vi "Main Panel.vi"() -> ()   [LabVIEW 2011]
uses:
  <vilib>/userdefined/High Color/IMAQdx.ctl
  <vilib>/vision/driver/NI_Vision_Acquisition_Software.lvlib
panel:
  out "Key Switch":bool
  out "Door Open":bool
  out "Flow Tank":dbl(slide) scale=0.0..100.0
  out "LCD Display":string
  out "Pump Irrigiation":bool
  out "Irrigation Empty Water":bool
  out "Hot Water On/Off?":bool
  out "AC/Heater On/Off?":bool
  out "What time you will be back?":dbl format="%#g"
  in  "STORE INFORMATIOn":bool
  out "Room2 Voice Recog":bool
  out "Room1 Voice Recog":bool
  out "Hot Water":bool
  out "Light Room2":bool
  out "Light Room1":bool
  in  "Hot Water":bool
  in  "Light Room2":bool
  in  "Light Room1":bool
  out "Manual AC Heater":bool
  in  "Manual Ac Heater":bool
  out "Fire Alarm":bool
  out "Manual Curtain":bool
  out "Curtain Open":bool
  out "Curtain close":bool
  in  "Close Curtain":bool
  in  "Open Curtain":bool
  in  "Manual Curtain":bool
  out "date":string
  out "time":string
  out "Solar Pos2":bool
  out "Solar Pos1":bool
  out "Light Intensity Pos2":dbl(knob) scale=0.0..100.0
  out "Light Intensity Pos1":dbl(knob) scale=0.0..100.0
  out "Water Temperature":dbl(slide) scale=0.0..100.0
  out "Temperature Inside":dbl(slide) scale=0.0..100.0
  out "Entree Light":bool
  out "RGB Door Led":bool
  out "Alarm Led":bool
  out "Low Level Water":bool
  out "Thief Alarm":bool
  out "Motion Detected":bool
  out "Dryer":bool
  out "Washing Machine":bool
  out "Heater":bool
  out "AC":bool
  in  "Restart Alarm":bool
  in  "Dryer":bool
  in  "AC":bool
  in  "Heater":bool
  in  "Washing Machine":bool
  out "WebCam":T1(plugin-control)
  in  "Exit":bool
  in  "Acess":bool
  out "Dor Lock/Unlock":bool
  in  "1":bool
  in  "2":bool
  in  "3":bool
  in  "4":bool
  in  "5":bool
  in  "6":bool
  in  "7":bool
  in  "8":bool
  in  "9":bool
  in  "0":bool
  out "Current":i32
  in  "0 2":bool
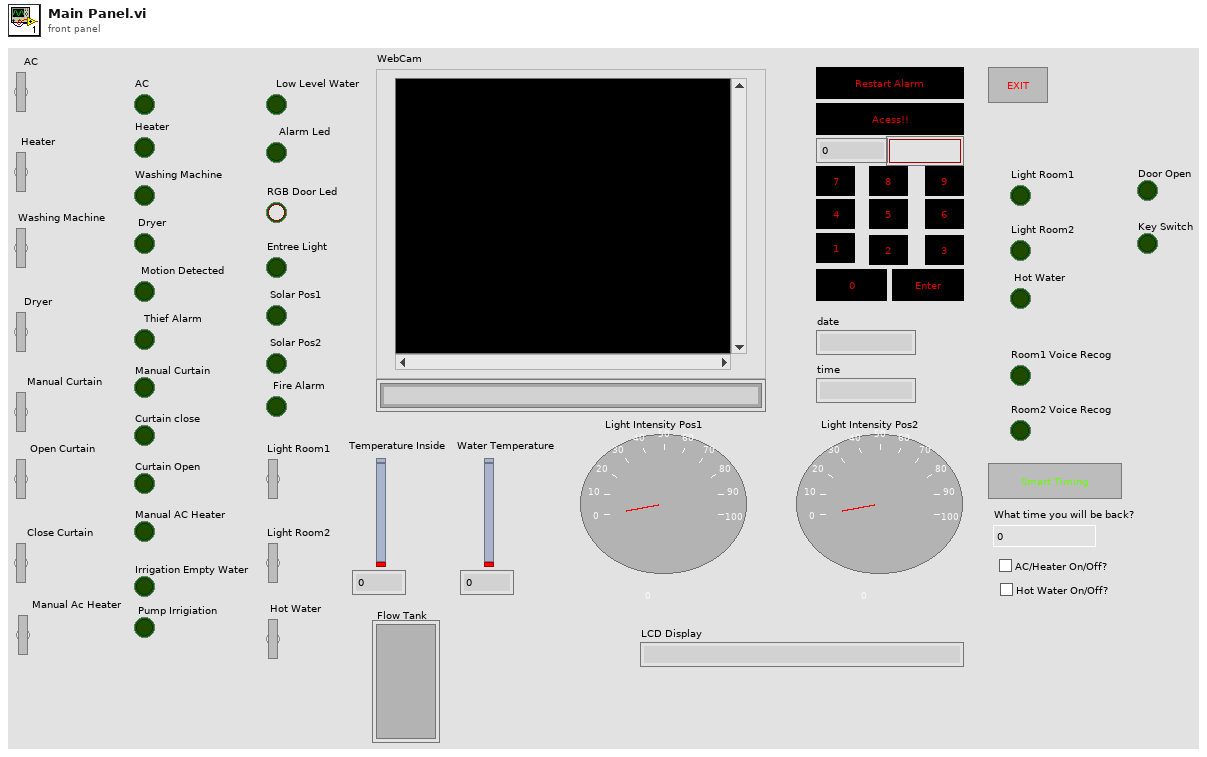
[diagram p1: front panel]
types:
  T1 = typedef "IMAQ Image.ctl" = refnum<image>
  T2 = typedef "IMAQdx.ctl" = refnum<k21>
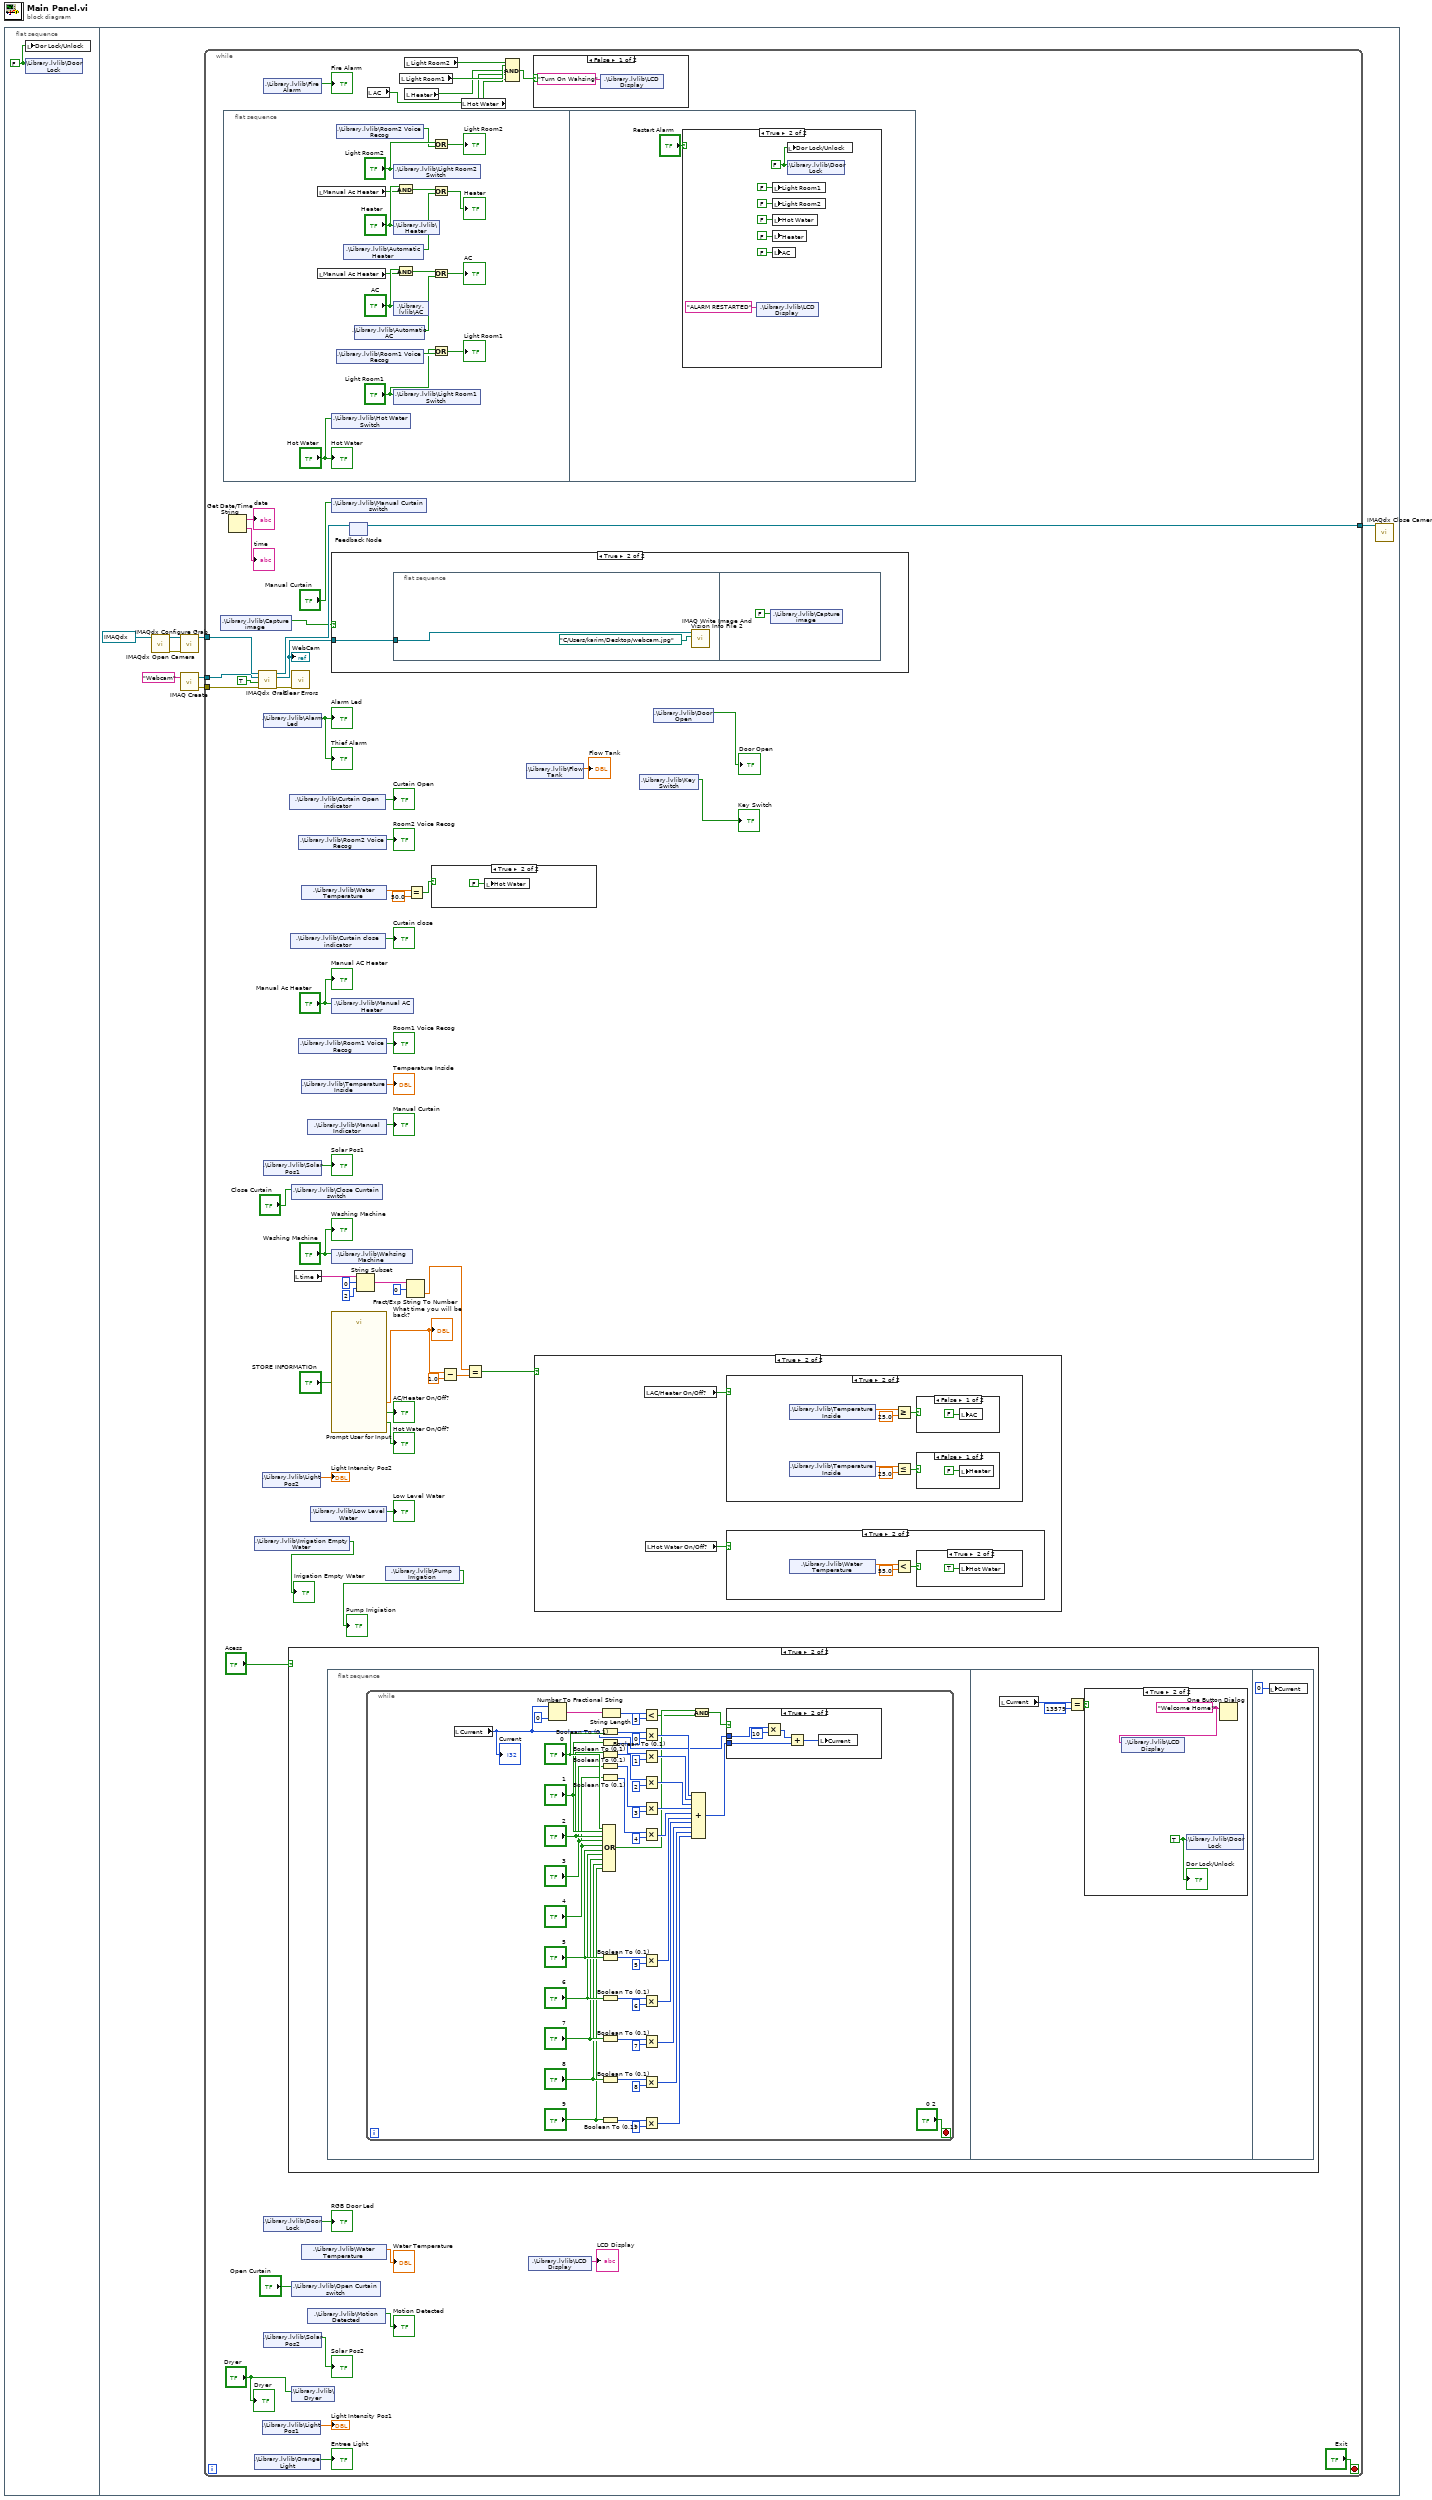
[diagram p0: block diagram]
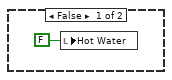
[diagram p5: hidden frame]
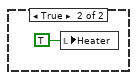
[diagram p7: hidden frame]
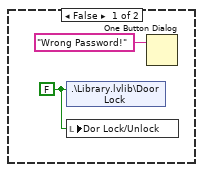
[diagram p13: hidden frame]
diagram:
  n1 = flat-sequence {
    frame #0 {
      w1 = FALSE ("Boolean")
      n2 = local write "Dor Lock/Unlock"(w1) -> ()
      n3 = shared-variable ".\\Library.lvlib\\Door Lock"(w1) -> ()  [unwired: 1 in, 1 out]
    }
    frame #1 {
      n4 = call <vilib>:"IMAQdx Open Camera.vi"("Session In"=T2 "cam0") -> ("error out"=w3:errorcluster, "Session Out"=w4:T2)  [unwired: 9 in]
      n5 = call <vilib>:"IMAQdx Configure Grab.vi"("error in"=w3, "Session In"=w4) -> ("Session Out"=w6:T2)  [unwired: 8 in, 1 out]
      n6 = call "IMAQ Create"("Image Name"="Webcam") -> ("New Image"=w5:T1, "error out"=w9:errorcluster)  [unwired: 4 in]
      n7 = while {
        tunnel: w5 -> [w69]
        tunnel: w6 -> [w72]
        tunnel: [w70] -> w7
        tunnel: w9 -> [w73]
        stop <- "Exit" stop-if-true
        n8 = shared-variable ".\\Library.lvlib\\Capture image"() -> (w63:bool)  [unwired: 1 in, 1 out]
        n9 = flat-sequence {
          frame #0 {
            n10 = local read "Manual Ac Heater"() -> (w93:bool)
            n11 = local read "Manual Ac Heater"() -> (w96:bool)
            n12 = shared-variable ".\\Library.lvlib\\Hot Water Switch"("Hot Water") -> ()  [unwired: 1 in, 1 out]
            n13 = shared-variable ".\\Library.lvlib\\Room2 Voice Recog"() -> (w104:bool)  [unwired: 1 in, 1 out]
            n14 = shared-variable ".\\Library.lvlib\\Room1 Voice Recog"() -> (w108:bool)  [unwired: 1 in, 1 out]
            n15 = shared-variable ".\\Library.lvlib\\Automatic Heater"() -> (w98:bool)  [unwired: 1 in, 1 out]
            n16 = shared-variable ".\\Library.lvlib\\Automatic AC"() -> (w101:bool)  [unwired: 1 in, 1 out]
            n17 = shared-variable ".\\Library.lvlib\\Light Room2 Switch"("Light Room2") -> ()  [unwired: 1 in, 1 out]
            n18 = shared-variable ".\\Library.lvlib\\Heater"("Heater") -> ()  [unwired: 1 in, 1 out]
            n19 = shared-variable ".\\Library.lvlib\\AC"("AC") -> ()  [unwired: 1 in, 1 out]
            n20 = shared-variable ".\\Library.lvlib\\Light Room1 Switch"("Light Room1") -> ()  [unwired: 1 in, 1 out]
            n21 = And(x="Heater", y=w93) -> (x .and. y?=w92:bool)
            n22 = And(x="AC", y=w96) -> (x .and. y?=w95:bool)
            n23 = Or(x="Light Room2", y=w104) -> (x .or. y?=→"Light Room2":bool)
            n24 = Or(x=w92, y=w98) -> (x .or. y?=→"Heater":bool)
            n25 = Or(x=w95, y=w101) -> (x .or. y?=→"AC":bool)
            n26 = Or(x="Light Room1", y=w108) -> (x .or. y?=→"Light Room1":bool)
            "Hot Water" <- "Hot Water"
          }
          frame #1 {
            n27 = case shown="True" "Restart Alarm" {
              frame False {
              }
              frame True {
                w116 = FALSE ("Boolean")
                n28 = shared-variable ".\\Library.lvlib\\LCD Display"("ALARM RESTARTED" ("LCD Display")) -> ()  [unwired: 1 in, 1 out]
                n29 = local write "Light Room1"(FALSE ("Light Room1")) -> ()
                n30 = local write "Light Room2"(FALSE ("Light Room2")) -> ()
                n31 = local write "Hot Water"(FALSE ("Hot Water")) -> ()
                n32 = local write "Heater"(FALSE ("Heater")) -> ()
                n33 = local write "AC"(FALSE ("AC")) -> ()
                n34 = local write "Dor Lock/Unlock"(w116) -> ()
                n35 = shared-variable ".\\Library.lvlib\\Door Lock"(w116) -> ()  [unwired: 1 in, 1 out]
              }
            }
          }
        }
        n36 = Get Date/Time String() -> (date string=→"date":string, time string=→"time":string)  [unwired: 3 in]
        n37 = shared-variable ".\\Library.lvlib\\Irrigation Empty Water"() -> (→"Irrigation Empty Water":bool)  [unwired: 1 in, 1 out]
        n38 = shared-variable ".\\Library.lvlib\\Orange Light"() -> (→"Entree Light":bool)  [unwired: 1 in, 1 out]
        n39 = call <vilib>:"IMAQdx Grab.vi"("error in"=w73, "Wait for Next Buffer? (Yes)"=TRUE, "Image In"=w69, "Session In"=w72) -> ("error out"=w64:errorcluster, "Image Out"=w66:T1, "Session Out"=w71:T2)  [unwired: 4 in, 1 out]
        "WebCam" <- w66
        n40 = shared-variable ".\\Library.lvlib\\Light Pos2"() -> (→"Light Intensity Pos2":dbl)  [unwired: 1 in, 1 out]
        n41 = shared-variable ".\\Library.lvlib\\Light Pos1"() -> (→"Light Intensity Pos1":dbl)  [unwired: 1 in, 1 out]
        n42 = shared-variable ".\\Library.lvlib\\Fire Alarm"() -> (→"Fire Alarm":bool)  [unwired: 1 in, 1 out]
        n43 = shared-variable ".\\Library.lvlib\\Alarm Led"() -> (→"Thief Alarm" →"Alarm Led":bool)  [unwired: 1 in, 1 out]
        n44 = shared-variable ".\\Library.lvlib\\Solar Pos1"() -> (→"Solar Pos1":bool)  [unwired: 1 in, 1 out]
        n45 = shared-variable ".\\Library.lvlib\\Door Lock"() -> (→"RGB Door Led":bool)  [unwired: 1 in, 1 out]
        n46 = shared-variable ".\\Library.lvlib\\Solar Pos2"() -> (→"Solar Pos2":bool)  [unwired: 1 in, 1 out]
        n47 = case shown="True" "Acess" {
          frame False {
          }
          frame True {
            n48 = flat-sequence {
              frame #0 {
                n49 = while {
                  stop <- "0 2" stop-if-true
                  n50 = local read "Current"() -> (w124:i32)
                  "Current" <- w124
                  n51 = Number To Fractional String(number=w124, precision (6)=i16 0) -> (F-format string=w122:string)  [unwired: 2 in]
                  n52 = Boolean To (0,1)(Boolean="0") -> (0, 1=w139:i16)
                  n53 = Boolean To (0,1)(Boolean="1") -> (0, 1=w150:i16)
                  n54 = Boolean To (0,1)(Boolean="2") -> (0, 1=w152:i16)
                  n55 = Boolean To (0,1)(Boolean="3") -> (0, 1=w154:i16)
                  n56 = Boolean To (0,1)(Boolean="4") -> (0, 1=w156:i16)
                  n57 = Boolean To (0,1)(Boolean="5") -> (0, 1=w158:i16)
                  n58 = Boolean To (0,1)(Boolean="6") -> (0, 1=w160:i16)
                  n59 = Boolean To (0,1)(Boolean="7") -> (0, 1=w162:i16)
                  n60 = Boolean To (0,1)(Boolean="8") -> (0, 1=w164:i16)
                  n61 = Boolean To (0,1)(Boolean="9") -> (0, 1=w166:i16)
                  n62 = String Length(string=w122) -> (length=w119:i32)
                  n63 = Compound Arithmetic op=OR("0", "1", "2", "3", "4", "5", "6", "7", "8", "9") -> (w121:bool)
                  n64 = Less?(x=w119, y=5) -> (x < y?=w117:bool)
                  n65 = Multiply(x=w139, y=i16 0) -> (x*y=w137:i16)
                  n66 = Multiply(x=w150, y=i16 1) -> (x*y=w148:i16)
                  n67 = Multiply(x=w152, y=i16 2) -> (x*y=w147:i16)
                  n68 = Multiply(x=w154, y=i16 3) -> (x*y=w146:i16)
                  n69 = Multiply(x=w156, y=i16 4) -> (x*y=w145:i16)
                  n70 = Multiply(x=w158, y=i16 5) -> (x*y=w144:i16)
                  n71 = Multiply(x=w160, y=i16 6) -> (x*y=w143:i16)
                  n72 = Multiply(x=w162, y=i16 7) -> (x*y=w142:i16)
                  n73 = Multiply(x=w164, y=i16 8) -> (x*y=w141:i16)
                  n74 = Multiply(x=w166, y=i16 9) -> (x*y=w140:i16)
                  n75 = Compound Arithmetic op=ADD(w137, w148, w147, w146, w145, w144, w143, w142, w141, w140) -> (w126:i16)
                  n76 = And(x=w121, y=w117) -> (x .and. y?=w120:bool)
                  n77 = case shown="True" w120 {
                    tunnel: w126 -> [_ w168]
                    tunnel: w124 -> [_ w167]
                    frame False {
                    }
                    frame True {
                      n78 = Multiply(x=w167, y=i16 10) -> (x*y=w171:i32)
                      n79 = Add(x=w171, y=w168) -> (x+y=w169:i32)
                      n80 = local write "Current"(w169) -> ()
                    }
                  }
                }
              }
              frame #1 {
                n81 = local read "Current"() -> (w174:i32)
                n82 = Equal?(x=w174, y=13579) -> (x = y?=w172:bool)
                n83 = case shown="True" w172 {
                  frame False {
                    w175 = FALSE ("Boolean")
                    n84 = shared-variable ".\\Library.lvlib\\Door Lock"(w175) -> ()  [unwired: 1 in, 1 out]
                    n85 = local write "Dor Lock/Unlock"(w175) -> ()
                    n86 = One Button Dialog(message="Wrong Password!") -> ()  [unwired: 1 in, 1 out]
                  }
                  frame True {
                    w178 = TRUE ("Boolean")
                    w177 = "Welcome Home!" ("message")
                    n87 = shared-variable ".\\Library.lvlib\\LCD Display"(w177) -> ()  [unwired: 1 in, 1 out]
                    n88 = shared-variable ".\\Library.lvlib\\Door Lock"(w178) -> ()  [unwired: 1 in, 1 out]
                    n89 = One Button Dialog(message=w177) -> ()  [unwired: 1 in, 1 out]
                    "Dor Lock/Unlock" <- w178
                  }
                }
              }
              frame #2 {
                n90 = local write "Current"(0 ("Current")) -> ()
              }
            }
          }
        }
        n91 = shared-variable ".\\Library.lvlib\\Curtain Open indicator"() -> (→"Curtain Open":bool)  [unwired: 1 in, 1 out]
        n92 = shared-variable ".\\Library.lvlib\\Curtain close indicator"() -> (→"Curtain close":bool)  [unwired: 1 in, 1 out]
        n93 = call <vilib>:"Clear Errors.vi"("error in (no error)"=w64) -> ()  [unwired: 6 in, 1 out]
        n94 = shared-variable ".\\Library.lvlib\\Close Currtain switch"("Close Curtain") -> ()  [unwired: 1 in, 1 out]
        n95 = shared-variable ".\\Library.lvlib\\Open Curtain switch"("Open Curtain") -> ()  [unwired: 1 in, 1 out]
        n96 = shared-variable ".\\Library.lvlib\\Dryer"("Dryer") -> ()  [unwired: 1 in, 1 out]
        n97 = local read "time"() -> (w26:string)
        n98 = shared-variable ".\\Library.lvlib\\Room2 Voice Recog"() -> (→"Room2 Voice Recog":bool)  [unwired: 1 in, 1 out]
        n99 = shared-variable ".\\Library.lvlib\\Room1 Voice Recog"() -> (→"Room1 Voice Recog":bool)  [unwired: 1 in, 1 out]
        n100 = shared-variable ".\\Library.lvlib\\Water Temperature"() -> (w37:dbl)  [unwired: 1 in, 1 out]
        n101 = shared-variable ".\\Library.lvlib\\Temperature Inside"() -> (→"Temperature Inside":dbl)  [unwired: 1 in, 1 out]
        n102 = shared-variable ".\\Library.lvlib\\Water Temperature"() -> (→"Water Temperature":dbl)  [unwired: 1 in, 1 out]
        n103 = shared-variable ".\\Library.lvlib\\Manual Indicator"() -> (→"Manual Curtain":bool)  [unwired: 1 in, 1 out]
        n104 = shared-variable ".\\Library.lvlib\\Motion Detected"() -> (→"Motion Detected":bool)  [unwired: 1 in, 1 out]
        n105 = shared-variable ".\\Library.lvlib\\Low Level Water"() -> (→"Low Level Water":bool)  [unwired: 1 in, 1 out]
        n106 = shared-variable ".\\Library.lvlib\\Manual Curtain switch"("Manual Curtain") -> ()  [unwired: 1 in, 1 out]
        n107 = case shown="True" w63 {
          tunnel: w66 -> [_ w180]
          frame False {
          }
          frame True {
            n108 = flat-sequence {
              tunnel: w180 -> [w181]
              frame #0 {
                n109 = call "IMAQ Write Image And Vision Info File 2"("File Path"=path "C:/Users/karim/Desktop/webcam.jpg", "Image"=w181) -> ()  [unwired: 8 in, 2 out]
              }
              frame #1 {
                n110 = shared-variable ".\\Library.lvlib\\Capture image"(FALSE ("Send Email")) -> ()  [unwired: 1 in, 1 out]
              }
            }
          }
        }
        n111 = shared-variable ".\\Library.lvlib\\Manual AC Heater"("Manual Ac Heater") -> ()  [unwired: 1 in, 1 out]
        n112 = shared-variable ".\\Library.lvlib\\Wahsing Machine"("Washing Machine") -> ()  [unwired: 1 in, 1 out]
        n113 = call "Prompt User for Input"("Enable"="STORE INFORMATIOn") -> ("Hot Water On/Off?"=→"Hot Water On/Off?":bool, "AC/Heater On/Off?"=→"AC/Heater On/Off?":bool, "What time you will be back?(24)"=w34:dbl)  [unwired: 14 in, 2 out]
        "What time you will be back?" <- w34
        n114 = feedback-in #1(w71) -> ()
        n115 = feedback #1() -> (w70:T2)  [unwired: 1 in]
        n116 = String Subset(string=w26, offset (0)=0, length (rest)=2 ("length (rest)")) -> (substring=w25:string)
        n117 = local read "AC"() -> (w12:bool)
        n118 = shared-variable ".\\Library.lvlib\\Pump Irrigation"() -> (→"Pump Irrigiation":bool)  [unwired: 1 in, 1 out]
        n119 = local read "Light Room1"() -> (w14:bool)
        n120 = local read "Light Room2"() -> (w15:bool)
        n121 = local read "Heater"() -> (w13:bool)
        n122 = Fract/Exp String To Number(string=w25, offset=0) -> (number=w28:dbl)  [unwired: 2 in, 1 out]
        n123 = Equal?(x=w37, y=50.0) -> (x = y?=w35:bool)
        n124 = case shown="True" w35 {
          frame False {
          }
          frame True {
            n125 = local write "Hot Water"(FALSE ("Hot Water")) -> ()
          }
        }
        n126 = Subtract(x=w34, y=1.0) -> (x-y=w30:dbl)
        n127 = local read "Hot Water"() -> (w11:bool)
        n128 = Equal?(x=w28, y=w30) -> (x = y?=w22:bool)
        n129 = Compound Arithmetic op=AND(w15, w14, w13, w12, w11) -> (w10:bool)
        n130 = shared-variable ".\\Library.lvlib\\Flow Tank"() -> (→"Flow Tank":dbl)  [unwired: 1 in, 1 out]
        n131 = shared-variable ".\\Library.lvlib\\LCD Display"() -> (→"LCD Display":string)  [unwired: 1 in, 1 out]
        n132 = case shown="False" w10 {
          frame False {
            n133 = shared-variable ".\\Library.lvlib\\LCD Display"("Turn On Wahsing" ("LCD Display")) -> ()  [unwired: 1 in, 1 out]
          }
          frame True {
          }
        }
        n134 = case shown="True" w22 {
          frame False {
          }
          frame True {
            n135 = local read "AC/Heater On/Off?"() -> (w75:bool)
            n136 = local read "Hot Water On/Off?"() -> (w76:bool)
            n137 = case shown="True" w75 {
              frame False {
              }
              frame True {
                n138 = shared-variable ".\\Library.lvlib\\Temperature Inside"() -> (w87:dbl)  [unwired: 1 in, 1 out]
                n139 = shared-variable ".\\Library.lvlib\\Temperature Inside"() -> (w83:dbl)  [unwired: 1 in, 1 out]
                n140 = Greater Or Equal?(x=w87, y=25.0) -> (x >= y?=w85:bool)
                n141 = Less Or Equal?(x=w83, y=25.0) -> (x <= y?=w82:bool)
                n142 = case shown="False" w85 {
                  frame False {
                    n143 = local write "AC"(FALSE ("AC")) -> ()
                  }
                  frame True {
                  }
                }
                n144 = case shown="False" w82 {
                  frame False {
                    n145 = local write "Heater"(FALSE ("Heater")) -> ()
                  }
                  frame True {
                    n146 = local write "Heater"(TRUE ("Heater")) -> ()
                  }
                }
              }
            }
            n147 = case shown="True" w76 {
              frame False {
              }
              frame True {
                n148 = shared-variable ".\\Library.lvlib\\Water Temperature"() -> (w79:dbl)  [unwired: 1 in, 1 out]
                n149 = Less?(x=w79, y=55.0) -> (x < y?=w77:bool)
                n150 = case shown="True" w77 {
                  frame False {
                    n151 = local write "Hot Water"(FALSE ("Hot Water")) -> ()
                  }
                  frame True {
                    n152 = local write "Hot Water"(TRUE ("Hot Water")) -> ()
                  }
                }
              }
            }
          }
        }
        n153 = shared-variable ".\\Library.lvlib\\Key Switch"() -> (→"Key Switch":bool)  [unwired: 1 in, 1 out]
        n154 = shared-variable ".\\Library.lvlib\\Door Open"() -> (→"Door Open":bool)  [unwired: 1 in, 1 out]
        "Washing Machine" <- "Washing Machine"
        "Dryer" <- "Dryer"
        "Manual AC Heater" <- "Manual Ac Heater"
      }
      n155 = call <vilib>:"IMAQdx Close Camera.vi"("Session In"=w7) -> ()  [unwired: 10 in, 1 out]
    }
  }
